vi "Faria-CSE360_Final_Project.vi"() -> ()   [LabVIEW 2020]
panel:
  out "Waveform Chart":dbl(graph)
  in  "Motion Detected":cluster{u32, u32}[](array[cluster])
  in  "Motion Done":cluster{u32, u32}[](array[cluster])
  out "Motion Detector LED":bool
  in  "High Temp":cluster{u32, u32}[](array[cluster])
  in  "Medium Temp":cluster{u32, u32}[](array[cluster])
  in  "Normal Temp":cluster{u32, u32}[](array[cluster])
  out "Temperature LED":bool
  out "Temperature":dbl
  out "Thermometer":dbl(slide) scale=70.0..110.0
  in  "VISA resource name":refnum<visa-resource-name>
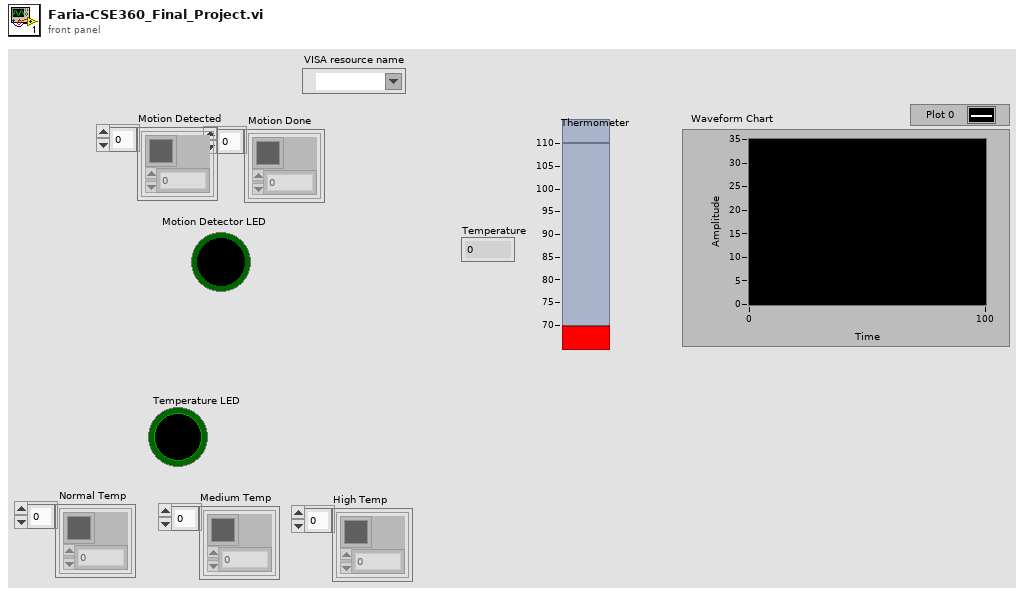
[diagram p1: front panel]
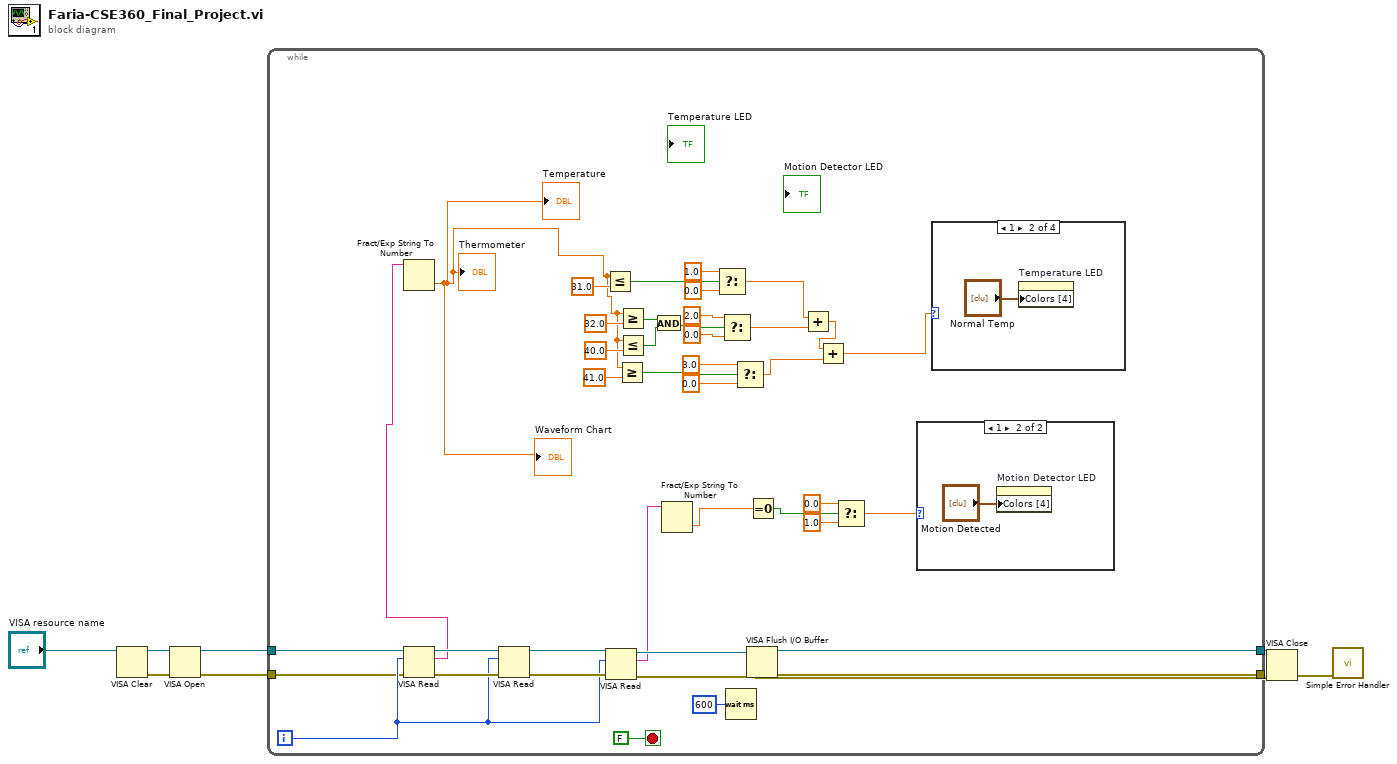
[diagram p0: block diagram]
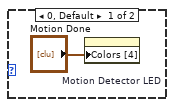
[diagram p2: hidden frame]
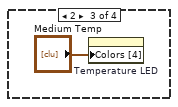
[diagram p4: hidden frame]
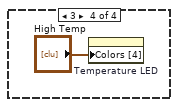
[diagram p5: hidden frame]
diagram:
  n1 = VISA Clear(VISA resource name="VISA resource name") -> (VISA resource name out=w8:refnum<visa-resource-name>, error out=w7:errorcluster)  [unwired: 1 in]
  n2 = VISA Open(error in (no error)=w7, VISA resource name=w8) -> (VISA resource name=w6:refnum<visa-resource-name>, error out=w5:errorcluster)  [unwired: 3 in]
  n3 = while {
    tunnel: w6 -> [w11]
    tunnel: w5 -> [w10]
    tunnel: [w49] -> w3
    tunnel: [w48] -> w4
    i -> [w13]
    stop <- FALSE stop-if-true
    n4 = VISA Read(VISA resource name=w11, byte count=w13, error in (no error)=w10) -> (VISA resource name out=w45:refnum<visa-resource-name>, read buffer=w23:string, error out=w44:errorcluster)  [unwired: 1 out]
    n5 = Fract/Exp String To Number(string=w23) -> (number=w9:dbl)  [unwired: 3 in, 1 out]
    "Thermometer" <- w9
    "Temperature" <- w9
    "Waveform Chart" <- w9
    n6 = VISA Read(VISA resource name=w45, byte count=w13, error in (no error)=w44) -> (VISA resource name out=w22:refnum<visa-resource-name>, error out=w14:errorcluster)  [unwired: 2 out]
    n7 = Less Or Equal?(x=w9, y=31.0) -> (x <= y?=w38:bool)
    n8 = VISA Read(VISA resource name=w22, byte count=w13, error in (no error)=w14) -> (VISA resource name out=w21:refnum<visa-resource-name>, read buffer=w19:string, error out=w20:errorcluster)  [unwired: 1 out]
    n9 = Greater Or Equal?(x=w9, y=41.0) -> (x >= y?=w29:bool)
    n10 = Greater Or Equal?(x=w9, y=32.0) -> (x >= y?=w40:bool)
    n11 = Less Or Equal?(x=w9, y=40.0) -> (x <= y?=w39:bool)
    n12 = And(x=w40, y=w39) -> (x .and. y?=w33:bool)
    n13 = Fract/Exp String To Number(string=w19) -> (number=w12:dbl)  [unwired: 3 in, 1 out]
    n14 = Select(t=1.0, s=w38, f=0.0) -> (s? t:f=w28:dbl)
    n15 = Select(t=2.0, s=w33, f=0.0) -> (s? t:f=w27:dbl)
    n16 = Wait (ms)(milliseconds to wait=u32 600) -> ()  [unwired: 1 out]
    n17 = Select(t=3.0, s=w29, f=0.0) -> (s? t:f=w25:dbl)
    n18 = VISA Flush I/O Buffer(VISA resource name=w21, error in (no error)=w20) -> (VISA resource name out=w49:refnum<visa-resource-name>, error out=w48:errorcluster)  [unwired: 1 in]
    n19 = Equal To 0?(x=w12) -> (x = 0?=w18:bool)
    n20 = Add(x=w28, y=w27) -> (x+y=w26:dbl)
    n21 = Add(x=w26, y=w25) -> (x+y=w24:dbl)
    n22 = Select(t=0.0, s=w18, f=1.0) -> (s? t:f=w15:dbl)
    n23 = case shown="1" w15 {
      frame 0, Default {
        n24 = property on="Motion Detector LED" class="Bool (strict)"("Colors [4]"="Motion Done") -> ()  [unwired: 2 in, 2 out]
      }
      frame 1 {
        n25 = property on="Motion Detector LED" class="Bool (strict)"("Colors [4]"="Motion Detected") -> ()  [unwired: 2 in, 2 out]
      }
    }
    n26 = case shown="1" w24 {
      frame 0, Default {
      }
      frame 1 {
        n27 = property on="Temperature LED" class="Bool (strict)"("Colors [4]"="Normal Temp") -> ()  [unwired: 2 in, 2 out]
      }
      frame 2 {
        n28 = property on="Temperature LED" class="Bool (strict)"("Colors [4]"="Medium Temp") -> ()  [unwired: 2 in, 2 out]
      }
      frame 3 {
        n29 = property on="Temperature LED" class="Bool (strict)"("Colors [4]"="High Temp") -> ()  [unwired: 2 in, 2 out]
      }
    }
  }
  n30 = VISA Close(VISA resource name=w3, error in (no error)=w4) -> (error out=w1:errorcluster)
  n31 = call <vilib>:"Simple Error Handler.vi"("error in (no error)"=w1) -> ()  [unwired: 4 in, 5 out]
